vi "getDamageQty.vi"(9 "Step":string, 10 "RCNo":string) -> (2 "Damage":i32)   [LabVIEW 2012]
uses:
  <vilib>/addons/database/Connection.llb/DB Tools Open Connec (Path).vi
  <vilib>/addons/database/Connection.llb/Conn Execute.vi
  <vilib>/addons/database/Recordset.llb/Rec Fetch Integer Data (R).vi
  <vilib>/addons/database/Recordset.llb/Rec Destroy - Connection.vi
  <vilib>/addons/database/NI_Database_API.lvlib
panel:
  out "error out":errorcluster
  out "concatenated string 2":string
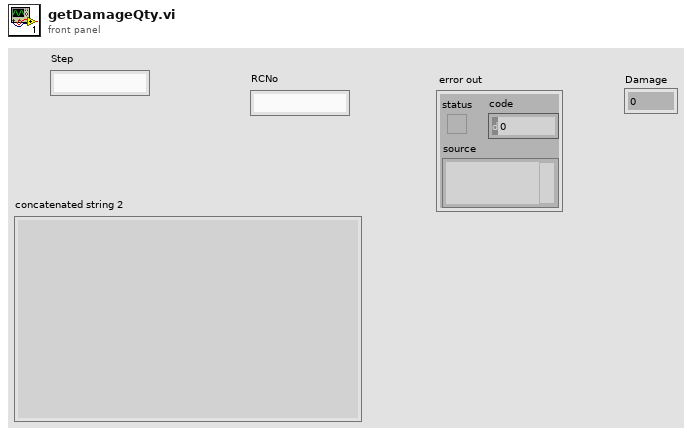
[diagram p1: front panel]
types:
  T1 = typedef "NI_Database_API.lvlib/Conn ObjectReference.ctl" = refnum<k1>
  T2 = typedef "NI_Database_API.lvlib/Rec ObjectReference.ctl" = refnum<k1>
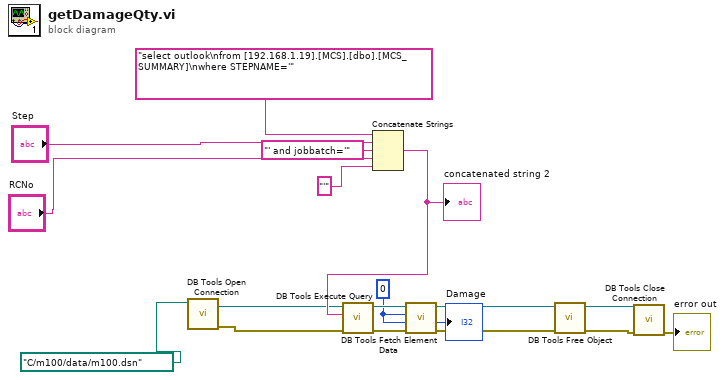
[diagram p0: block diagram]
diagram:
  w5 = 0
  n1 = call-poly <vilib>:"DB Tools Open Connection.vi"("connection information"=path "C:/m100/data/m100.dsn") -> ("error out"=w10:errorcluster, "connection reference"=w11:T1)  [unwired: 7 in]
  n2 = Concatenate Strings("select outlook\nfrom [192.168.1.19].[MCS].[dbo].[MCS_SUMMARY]\nwhere STEPNAME='" ("string"), "Step", "' and jobbatch='" ("string"), "RCNo", "'" ("string")) -> (w17:string)
  "concatenated string 2" <- w17
  n3 = call-poly <vilib>:"DB Tools Execute Query.vi"("error in (no error)"=w10, "SQL query"=w17, "connection reference"=w11) -> ("error out"=w14:errorcluster, "recordset reference"=w16:T2)  [unwired: 5 in]
  n4 = call-poly <vilib>:"DB Tools Fetch Element Data.vi"("error in (no error)"=w14, "type"=w5, "column index"=w5, "recordset reference"=w16) -> ("error out"=w13:errorcluster, "data"=→"Damage":i32, "recordset reference out"=w15:T2)  [unwired: 3 in]
  n5 = call-poly <vilib>:"DB Tools Free Object.vi"("error in (no error)"=w13, "recordset reference"=w15) -> ("error out"=w2:errorcluster, "connection reference"=w3:T1)  [unwired: 8 in]
  n6 = call <vilib>:"DB Tools Close Connection.vi"("error in (no error)"=w2, "connection reference"=w3) -> ("error out"=→"error out":errorcluster)  [unwired: 5 in]
